vi "replaceYearMonthToken.vi"(8 "error in (no error)":errorcluster, 10 "Query In":string, 11 "WhichMonth in":refnum<class "WhichMonth.lvclass">) -> (0 "error out":errorcluster, 2 "Query Out":string, 3 "WhichMonth out":refnum<class "WhichMonth.lvclass">)   [LabVIEW 2018, in "WhichMonth.lvclass"]
uses:
  WhichMonth.lvclass
  WhichMonth.lvclass/WhichMonth.ctl
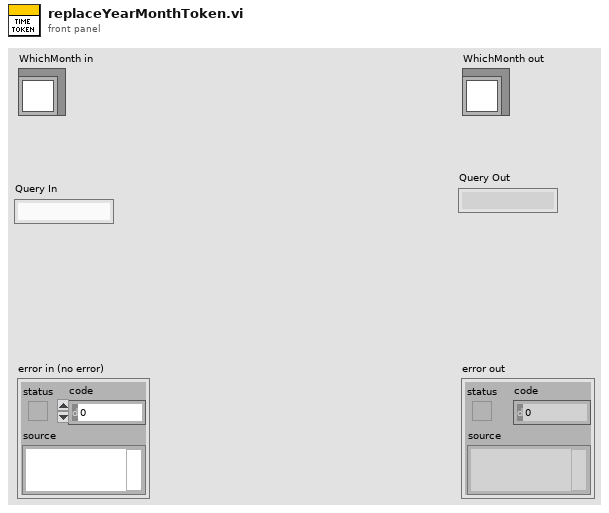
[diagram p1: front panel]
types:
  T1 = typedef "WhichMonth.lvclass/Month.ctl" = enum16{"January", "February", "March", "April", "May", "June", "July", "August", "September", "October", "November", "December"}
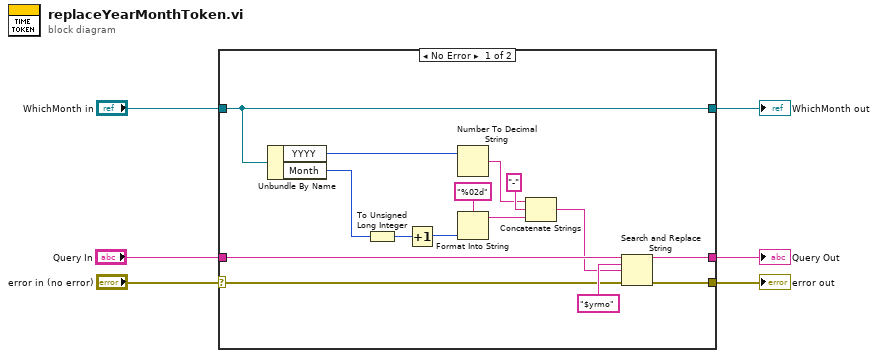
[diagram p0: block diagram]
diagram:
  n1 = case shown="No Error" "error in (no error)" {
    selector: "error in (no error)" -> [w9 w24]
    tunnel: [w7 w24] -> w5
    tunnel: [w13 w23] -> w3
    tunnel: "WhichMonth in" -> [w13 w23]
    tunnel: "Query In" -> [w12 w22]
    tunnel: [w8 w22] -> w1
    frame No Error {
      n2 = Unbundle By Name(w13) -> ("YYYY"=w15:i32, "Month"=w14:T1)
      n3 = To Unsigned Long Integer(number=w14) -> (unsigned 32bit integer=w17:u32)
      n4 = Increment(x=w17) -> (x+1=w16:u32)
      n5 = Number To Decimal String(number=w15) -> (decimal integer string=w18:string)  [unwired: 1 in]
      n6 = Format Into String(format string="%02d" ("string"), w16) -> (resulting string=w20:string)  [unwired: 2 in, 1 out]
      n7 = Concatenate Strings(w18, "-" ("string"), w20) -> (w10:string)
      n8 = Search and Replace String(input string=w12, search string="$yrmo", replace string=w10, error in=w9) -> (result string=w8:string, error out=w7:errorcluster)  [unwired: 4 in, 2 out]
    }
    frame Error {
    }
  }
  "error out" <- w5
  "WhichMonth out" <- w3
  "Query Out" <- w1
